vi "TreeViewAddItemIndent.vi"(0 "TreeControl in":refnum<vi>, 1 "Indentation":i32, 5 "Left Cell String":string, 7 "Child Text":string[](array[string]), 9 "Tag":string, 11 "error in (no error)":errorcluster, 12 "Symbol Index":i32, 13 "Background Color":u32(colorbox)=16777215, 14 "Bold Font":bool) -> (4 "TreeControl out":refnum<vi>, 10 "Tag out":string, 15 "error out":errorcluster)   [LabVIEW 2019, in "VIPropertyPicker.lvlib"]
uses:
  VIPropertyPicker.lvlib
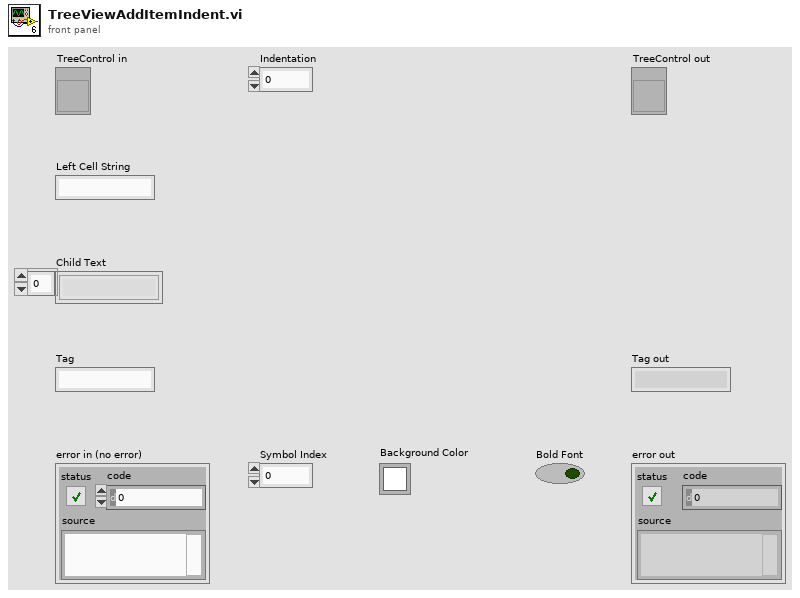
[diagram p1: front panel]
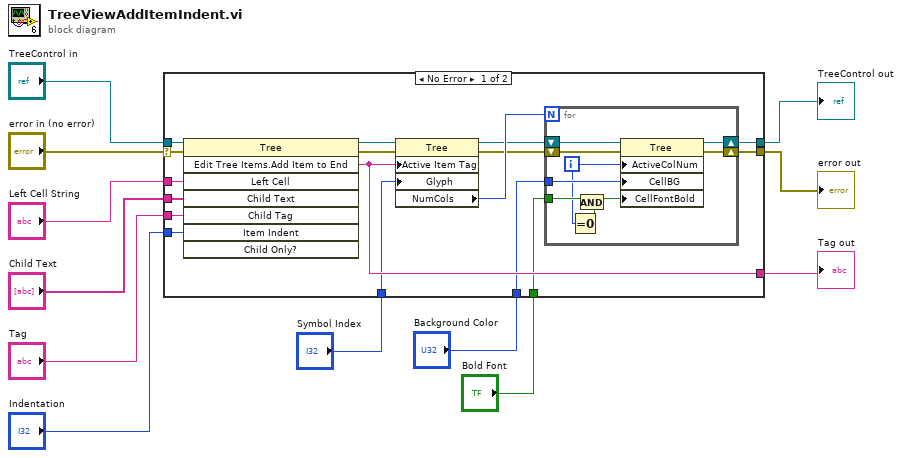
[diagram p0: block diagram]
diagram:
  n1 = case shown="No Error" "error in (no error)" {
    selector: "error in (no error)" -> [w13 w41]
    tunnel: [w29 w41] -> w12
    tunnel: [w25 w39] -> w11
    tunnel: "Left Cell String" -> [w22 w39]
    tunnel: "TreeControl in" -> [w21 w40]
    tunnel: "Child Text" -> [w20 _]
    tunnel: "Tag" -> [w19 _]
    tunnel: "Indentation" -> [w18 _]
    tunnel: "Symbol Index" -> [w17 _]
    tunnel: "Background Color" -> [w16 _]
    tunnel: [w15 w40] -> w3
    tunnel: "Bold Font" -> [w14 _]
    frame No Error {
      n2 = invoke class="Tree" method="Edit Tree Items.Add Item to End"(reference=w21, error in=w13, "Left Cell"=w22, "Child Text"=w20, "Child Tag"=w19, "Item Indent"=w18) -> (reference out=w23:refnum<vi>, error out=w24:errorcluster, "Edit Tree Items:Add Item to End"=w25:string)  [unwired: 2 in, 5 out]
      n3 = property class="Tree"(reference=w23, error in=w24, "Active Item Tag"=w25, "Glyph"=w17) -> (reference out=w26:refnum<vi>, error out=w27:errorcluster, "NumCols"=w28:u32)
      n4 = for {
        N: w28 -> [_]
        shift-right: [w36] -> w29
        shift-left: w27 -> [w37]
        tunnel: w16 -> [w35]
        shift-right: [w34] -> w15
        shift-left: w26 -> [w38]
        tunnel: w14 -> [w33]
        i -> [w31]
        n5 = Equal To 0?(x=w31) -> (x = 0?=w30:bool)
        n6 = And(x=w33, y=w30) -> (x .and. y?=w32:bool)
        n7 = property class="Tree"(reference=w38, error in=w37, "ActiveColNum"=w31, "CellBG"=w35, "CellFontBold"=w32) -> (reference out=w34:refnum<vi>, error out=w36:errorcluster)
      }
    }
    frame Error {
    }
  }
  "error out" <- w12
  "TreeControl out" <- w3
  "Tag out" <- w11
